vi "Facade 1.vi"(0 "Data In":T4, 2 "Display State In":T2, 3 "Container State":T3) -> (6 "Data Out":T4, 7 "Display State Out":T2, 8 "Action":T1)   [LabVIEW 2018, in "Start Button.xctl"]
uses:
  Start Button.xctl
  Data 1.ctl
  <vilib>/_xctls/Container State.ctl
  State 1.ctl
  <vilib>/_xctls/Action.ctl
  <vilib>/_xctls/XControlSupport.lvlib
panel:
  in  "INICIAR":bool
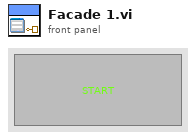
[diagram p1: front panel]
types:
  T1 = typedef "XControlSupport.lvlib/Action.ctl" = cluster{"Data Changed?":bool, "State Changed?":bool, "Action Name":string}
  T2 = typedef "Start Button.xctl/State 1.ctl" = cluster{"Numeric":dbl}
  T3 = typedef "XControlSupport.lvlib/Container State.ctl" = cluster{"Indicator?":bool, "Run Mode?":bool, " Refnum":refnum<vi>}
  T4 = typedef "Start Button.xctl/Data 1.ctl" = dbl
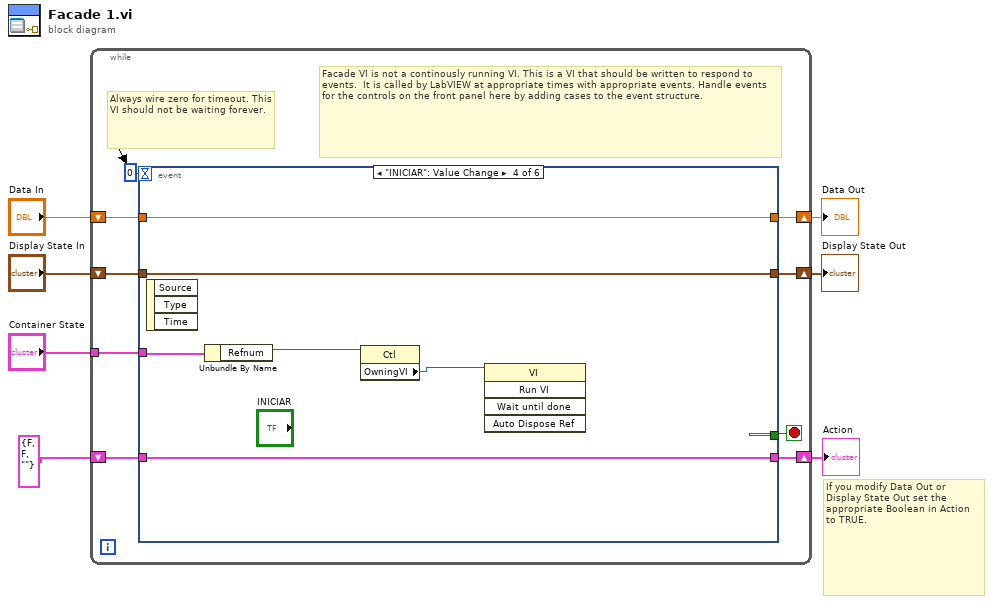
[diagram p0: block diagram]
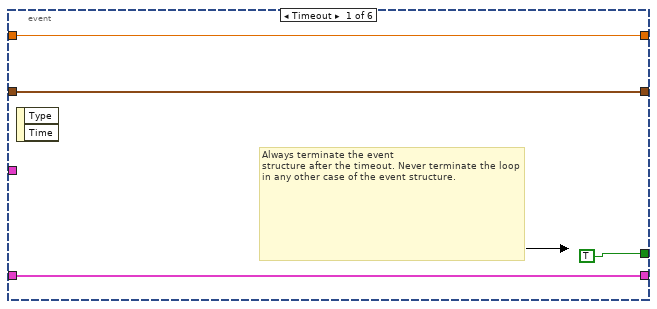
[diagram p2: hidden frame]
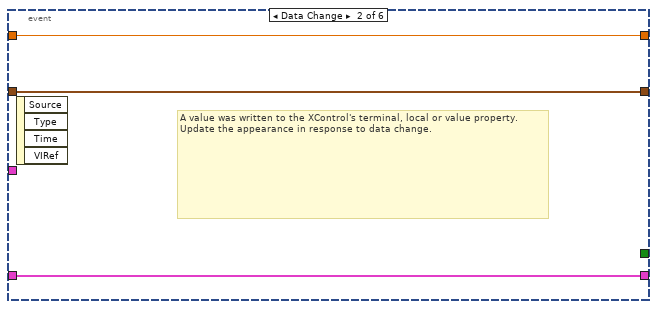
[diagram p3: hidden frame]
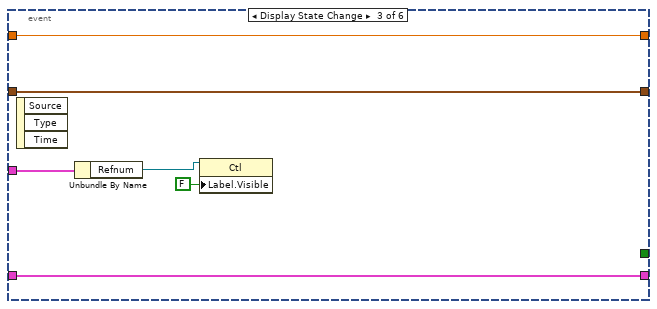
[diagram p4: hidden frame]
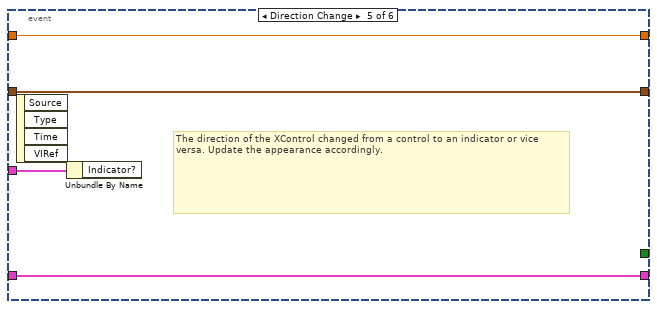
[diagram p5: hidden frame]
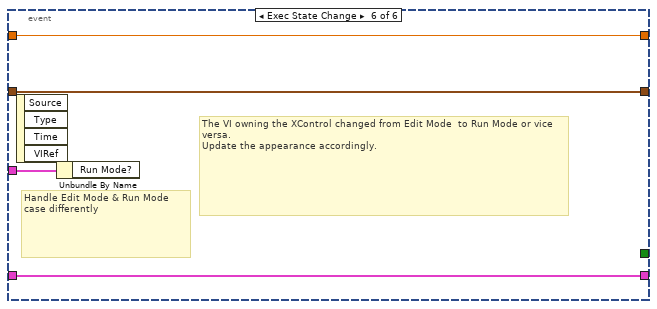
[diagram p6: hidden frame]
diagram:
  # "If you modify Data Out or\nDisplay State Out set the\nappropriate Boolean in Action\nto TRUE."
  n1 = while {
    shift-right: [w15] -> w4
    shift-left: "Display State In" -> [w16]
    tunnel: "Container State" -> [w12]
    shift-right: [w10] -> w7
    shift-left: "Data In" -> [w11]
    shift-right: [w8] -> w2
    shift-left: T1 {"Data Changed?"=FALSE, "State Changed?"=FALSE, "Action Name"=""} ("Action") -> [w9]
    stop <- w14 stop-if-true
    # "Facade VI is not a continously running VI. This is a VI that should be written to respond to events.  It is called by LabVIEW at appropriate times with appropriate events. Handle events for the controls on the front panel here by adding cases to the event structure."
    # "Always wire zero for timeout. This\nVI should not be waiting forever."
    n2 = event shown="[3] \"INICIAR\": Value Change" {
      selector: _ -> [_ _ _ _ _ _]
      dyn-events: _ -> [_ _ _ _ _ _]
      timeout: 0 -> [_ _ _ _ _ _]
      tunnel: w16 -> [w18 w22 w29 w35 w38 w42]
      tunnel: [w18 w22 w29 w35 w38 w42] -> w15
      tunnel: [TRUE _ _ _ _ _] -> w14
      tunnel: w12 -> [_ _ w26 w32 w39 w43]
      tunnel: w11 -> [w17 w23 w28 w34 w37 w41]
      tunnel: [w17 w23 w28 w34 w37 w41] -> w10
      tunnel: [w19 w21 w27 w33 w36 w40] -> w8
      tunnel: w9 -> [w19 w21 w27 w33 w36 w40]
      event Timeout {
        # "Always terminate the event\nstructure after the timeout. Never terminate the loop in any other case of the event structure."
        n3 = event-data() -> ()  [unwired: 1 in, 2 out]
      }
      event Data Change {
        # "A value was written to the XControl's terminal, local or value property.\nUpdate the appearance in response to data change."
        n4 = event-data() -> ()  [unwired: 1 in, 4 out]
      }
      event Display State Change {
        n5 = event-data() -> ()  [unwired: 1 in, 3 out]
        n6 = Unbundle By Name(w26) -> ("Refnum"=w25:refnum<vi>)
        n7 = property class="Ctl"(reference=w25, "Label.Visible"=FALSE) -> ()  [unwired: 1 in, 2 out]
      }
      event "INICIAR": Value Change {
        n8 = event-data() -> ()  [unwired: 1 in, 3 out]
        n9 = Unbundle By Name(w32) -> ("Refnum"=w31:refnum<vi>)
        n10 = property class="Ctl"(reference=w31) -> ("OwningVI"=w30:refnum<vi>)  [unwired: 1 in, 2 out]
        n11 = invoke class="VI" method="Run VI"(reference=w30) -> ()  [unwired: 4 in, 5 out]
      }
      event Direction Change {
        # "The direction of the XControl changed from a control to an indicator or vice versa. Update the appearance accordingly."
        n12 = event-data() -> ()  [unwired: 1 in, 4 out]
        n13 = Unbundle By Name(w39) -> ()  [unwired: 1 out]
      }
      event Exec State Change {
        # "The VI owning the XControl changed from Edit Mode  to Run Mode or vice versa.\nUpdate the appearance accordingly."
        # "Handle Edit Mode & Run Mode\ncase differently"
        n14 = event-data() -> ()  [unwired: 1 in, 4 out]
        n15 = Unbundle By Name(w43) -> ()  [unwired: 1 out]
      }
    }
  }
  "Display State Out" <- w4
  "Data Out" <- w7
  "Action" <- w2
